vi "Update Frame Trees.vi"(8 "error in":errorcluster, 9 "acyclic frames tree":refnum<vi>, 10 "major minor frames tree":refnum<vi>, 11 "Node Ptr":T1 format="%.0x") -> (0 "error out":errorcluster, 3 "Node Ptr out":T1 format="%.0x")   [LabVIEW 2020, in "AIM MIL-STD-1553 System Explorer.lvlib" / "Implementation.lvlib"]
uses:
  Implementation.lvlib
  <vilib>/NI VeriStand/Custom Device API/Custom Device API.lvlib
  Scripting/AIM MIL-STD-1553 Scripting.lvlib
  <vilib>/NI VeriStand/Custom Device API/Custom Device Item Ref.ctl
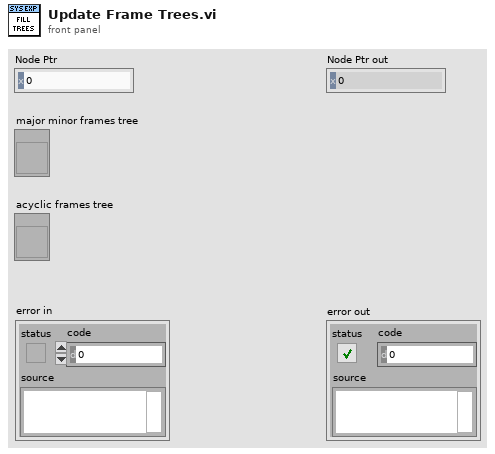
[diagram p1: front panel]
types:
  T1 = typedef "Custom Device API.lvlib/Custom Device Item Ref.ctl" = u64
  T2 = typedef "Minor Frame Definition.ctl" = cluster{"name":string, "messages":string[]}
  T3 = typedef "Major Frame Definition.ctl" = cluster{"name":string, "minor frames":string[]}
  T4 = typedef "Acyclic Frame Definition.ctl" = cluster{"name":string, "messages":string[]}
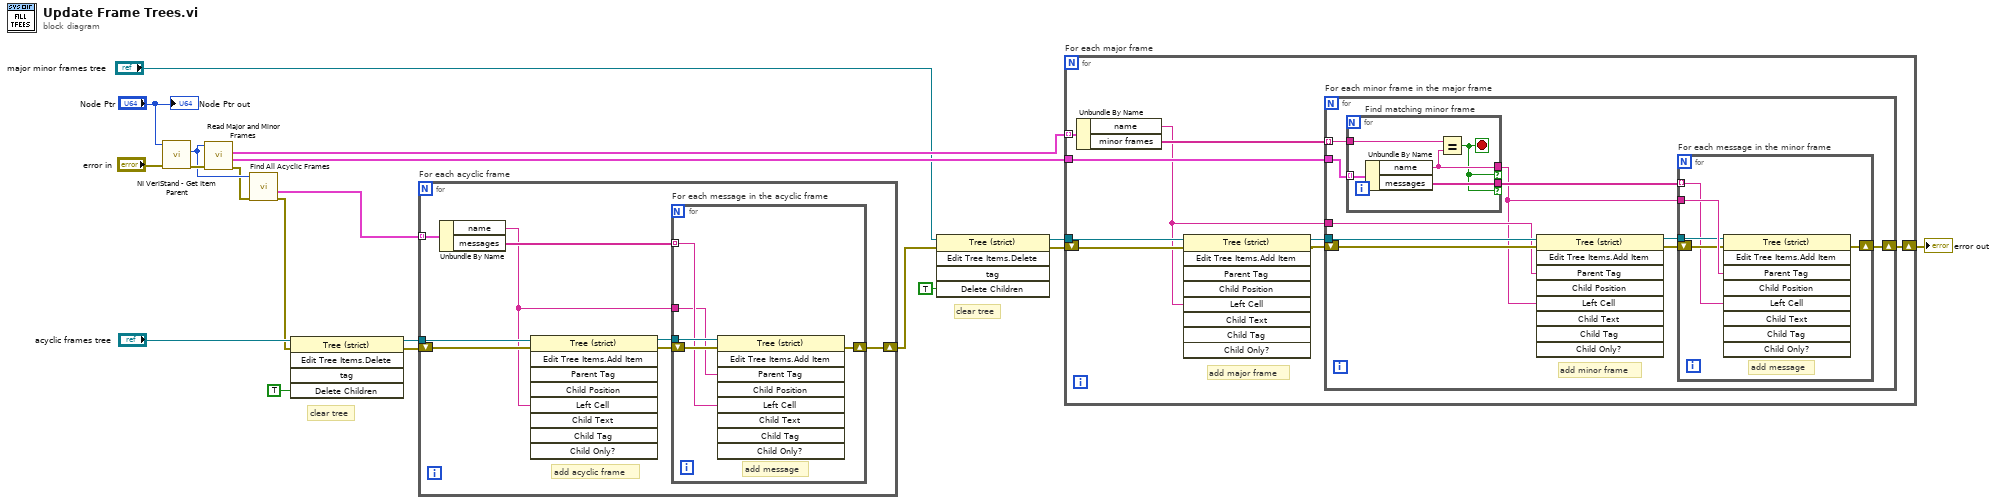
[diagram p0: block diagram]
diagram:
  # "clear tree"
  # "clear tree"
  n1 = call <vilib>:"NI VeriStand - Get Item Parent.vi"("error in (no error)"="error in", "Item Ref in"="Node Ptr") -> ("error out"=w18:errorcluster, "Parent Ref"=w11:T1)  [unwired: 6 in, 2 out]
  n2 = call "Read Major and Minor Frames.vi"("error in"=w18, "port"=w11) -> ("error out"=w3:errorcluster, "minor frames"=w16:T2[], "major frames"=w17:T3[])  [unwired: 6 in, 1 out]
  n3 = call "Find All Acyclic Frames.vi"("error in"=w3, "port"=w11) -> ("error out"=w8:errorcluster, "acyclic frames"=w5:T4[])  [unwired: 6 in, 2 out]
  n4 = invoke class="Tree (strict)" method="Edit Tree Items.Delete"(reference="acyclic frames tree", error in=w8, "Delete Children"=TRUE ("Delete Children?")) -> (reference out=w6:refnum<vi>, error out=w7:errorcluster)  [unwired: 2 in, 3 out]
  n5 = for "For each acyclic frame" {
    tunnel: w6 -> [w26]
    shift-right: [w25] -> w4
    shift-left: w7 -> [w27]
    tunnel: w5 -> [w24] mode=indexing
    # "add acyclic frame"
    n6 = Unbundle By Name(w24) -> ("name"=w20:string, "messages"=w21:string[])
    n7 = invoke class="Tree (strict)" method="Edit Tree Items.Add Item"(reference=w26, error in=w27, "Left Cell"=w20) -> (reference out=w23:refnum<vi>, error out=w22:errorcluster)  [unwired: 6 in, 7 out]
    n8 = for "For each message in the acyclic frame" {
      tunnel: w23 -> [w32]
      tunnel: w21 -> [w30] mode=indexing
      shift-right: [w29] -> w25
      shift-left: w22 -> [w31]
      tunnel: w20 -> [w28]
      # "add message"
      n9 = invoke class="Tree (strict)" method="Edit Tree Items.Add Item"(reference=w32, error in=w31, "Parent Tag"=w28, "Left Cell"=w30) -> (error out=w29:errorcluster)  [unwired: 5 in, 8 out]
    }
  }
  n10 = invoke class="Tree (strict)" method="Edit Tree Items.Delete"(reference="major minor frames tree", error in=w4, "Delete Children"=TRUE ("Delete Children?")) -> (reference out=w12:refnum<vi>, error out=w13:errorcluster)  [unwired: 2 in, 3 out]
  n11 = for "For each major frame" {
    tunnel: w17 -> [w41] mode=indexing
    tunnel: w16 -> [w40]
    tunnel: w12 -> [w38]
    shift-right: [w33] -> w2
    shift-left: w13 -> [w39]
    # "add major frame"
    n12 = Unbundle By Name(w41) -> ("name"=w36:string, "minor frames"=w37:string[])
    n13 = invoke class="Tree (strict)" method="Edit Tree Items.Add Item"(reference=w38, error in=w39, "Left Cell"=w36) -> (reference out=w35:refnum<vi>, error out=w34:errorcluster)  [unwired: 6 in, 7 out]
    n14 = for "For each minor frame in the major frame" {
      tunnel: w37 -> [w50] mode=indexing
      tunnel: w40 -> [w51]
      tunnel: w36 -> [w47]
      tunnel: w35 -> [w49]
      shift-right: [w42] -> w33
      shift-left: w34 -> [w48]
      # "add minor frame"
      n15 = for "Find matching minor frame" {
        tunnel: w51 -> [w61] mode=indexing
        tunnel: w50 -> [w60]
        tunnel: [w59] -> w43 if=w57
        tunnel: [w58] -> w44 if=w57
        stop <- w57 stop-if-true
        n16 = Unbundle By Name(w61) -> ("name"=w59:string, "messages"=w58:string[])
        n17 = Equal?(x=w60, y=w59) -> (x = y?=w57:bool)
      }
      n18 = invoke class="Tree (strict)" method="Edit Tree Items.Add Item"(reference=w49, error in=w48, "Parent Tag"=w47, "Left Cell"=w43) -> (reference out=w46:refnum<vi>, error out=w45:errorcluster)  [unwired: 5 in, 7 out]
      n19 = for "For each message in the minor frame" {
        tunnel: w46 -> [w55]
        tunnel: w44 -> [w53] mode=indexing
        tunnel: w43 -> [w56]
        shift-right: [w52] -> w42
        shift-left: w45 -> [w54]
        # "add message"
        n20 = invoke class="Tree (strict)" method="Edit Tree Items.Add Item"(reference=w55, error in=w54, "Parent Tag"=w56, "Left Cell"=w53) -> (error out=w52:errorcluster)  [unwired: 5 in, 8 out]
      }
    }
  }
  "error out" <- w2
  "Node Ptr out" <- "Node Ptr"
